vi "DataReceiver.vi"() -> ()   [LabVIEW 2015]
panel:
  out "Waveform Graph":sgl[][](graph)
  in  "stop":bool
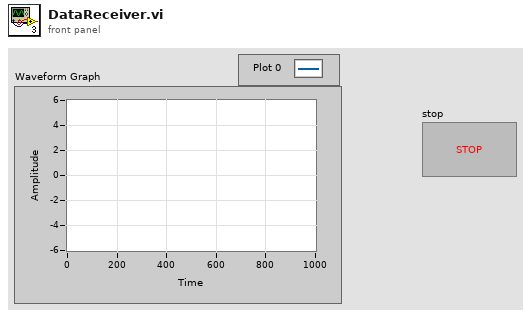
[diagram p1: front panel]
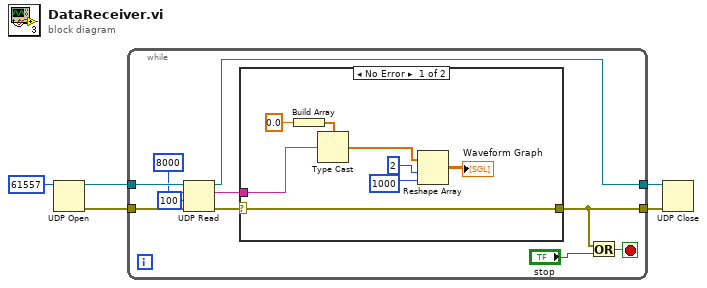
[diagram p0: block diagram]
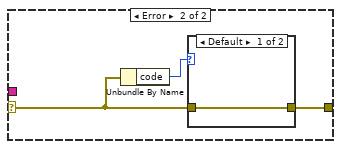
[diagram p2: hidden frame]
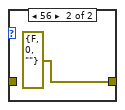
[diagram p3: hidden frame]
diagram:
  n1 = UDP Open(11:u16 61557 ("port")) -> (port=w5:refnum<k16>, 0:w4:errorcluster)  [unwired: 4 in, 1 out]
  n2 = while {
    tunnel: w5 -> [w15]
    tunnel: w4 -> [w14]
    tunnel: [w12] -> w3
    tunnel: [w9] -> w2
    stop <- w10 stop-if-true
    n3 = UDP Read(connection ID=w15, max size (548)=8000, timeout ms (25000)=100, 8:w14) -> (data out=w11:string, error out=w13:errorcluster, 3:w12:refnum<k16>)  [unwired: 2 out]
    n4 = case shown="No Error" w13 {
      selector: w13 -> [w17 w24]
      tunnel: [w17 w25] -> w9
      tunnel: w11 -> [w18 _]
      frame No Error {
        n5 = Build Array(sgl 0.0 ("element")) -> (w23:sgl[])
        n6 = Type Cast(type=w23, x=w18) -> (*(type *) &x=w22:sgl[])
        n7 = Reshape Array(w22, 2 ("dimension size"), 1000 ("dimension size")) -> (→"Waveform Graph":sgl[][])
      }
      frame Error {
        n8 = Unbundle By Name(w24) -> ("code"=w26:i32)
        n9 = case shown="Default" w26 {
          tunnel: [w27 errorcluster {"status"=FALSE, "code"=0, "source"=""} ("error constant")] -> w25
          tunnel: w24 -> [w27 _]
          frame Default {
          }
          frame 56 {
          }
        }
      }
    }
    n10 = Or(x=w9, y="stop") -> (x .or. y?=w10:bool)
  }
  n11 = UDP Close(connection ID=w3, 8:w2) -> ()  [unwired: 2 out]
